vi "normal_FGV.vi"(2 "data":string) -> (7 "data":string)   [LabVIEW 2015]
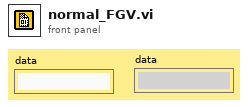
[diagram p1: front panel]
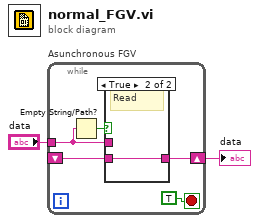
[diagram p0: block diagram]
diagram:
  n1 = while "Asunchronous FGV" {
    tunnel: "data" -> [w5]
    shift-right: [w6] -> w1
    shift-left: _ -> [w3]
    stop <- TRUE stop-if-true
    n2 = Empty String/Path?(string/path=w5) -> (empty?=w4:bool)
    n3 = case shown="True" w4 {
      tunnel: w5 -> [w8 _]
      tunnel: [w8 w9] -> w6
      tunnel: w3 -> [_ w9]
      frame False {
        # "Write"
      }
      frame True {
        # "Read"
      }
    }
  }
  "data" <- w1
